vi "Phase Plots.vi"(4 "Impulse Positions":T3(array[cluster]) {"Amplitude offset" format="%.2f"}, 5 "Data Output":T4 {"Data Channels" format="%.2f"}, 7 "desacc":T1={"Threshold 1 [Acc]"=0.0, "Threshold 2 [% of TH1]"=0, "tolerance"=2, "Search WD "=0.05757575757575758, " always use TH2"=TRUE, "Range"=3.0303030303030303, "Max time"=50.0, "Min time"=1.0, "Velocity Threshold"=3.0303030303030303} {"Velocity Threshold" scale=0.0..5.0; "Range" scale=0.0..5.0; "Search WD" scale=0.0..0.3; "tolerance" scale=0.0..10.0; "Threshold 2 [% of TH1]" scale=0.0..100.0; "Threshold 1 [Acc]" scale=1.0..20000.0}) -> ()   [LabVIEW 2016]
uses:
  <vilib>/Analysis/baseanly.llb/Mean (DBL).vi
  comm/impulse/impulse functions.lvlib
  <vilib>/Analysis/NI_AALPro.lvlib
  <vilib>/Analysis/NI_AALBase.lvlib
panel:
  out "Angle Error":dbl format="%#_4g"
  out "Angle":dbl format="%#_4g"
  out "Slope":dbl
  out "Const":dbl
  out "Plane Equation":T2 {"Standard Deviation" format="%.6f"; "Z Slope" format="%.6f"; "Y Slope" format="%.6f"; "Offset" format="%.6f"}
  in  "Recalculate":bool
  in  "Horizontal Channel":u16(ring)=27
  in  "Vertical Channel":u16(ring)=27
  in  "Torsion Channel":u16(ring)=27
  in  "Fixed Absicca":bool
  in  "Fixed Ordinate":bool
  out "Phase Plot":cluster{dbl[], dbl[]}[](graph)
  in  "stop":bool
  in  "Off     Gain Inv         Absicca                         Off    Gain  Inv         Ordinate             Col  Sac    Plane          Data Range":T5(array[cluster])=[{"Color Box"=16777222, "Channel 1"=27, "inv 1"=FALSE, "Sac"=FALSE, "Offset 1"=0.0, "Gain 1"=1.0, "channel 2"=27, "Data From"=0, "Impulse Plane"=enum."Yaw", "inv 2"=FALSE, "Offset 2"=0.0, "Gain 2"=1.0}, {"Color Box"=3381759, "Channel 1"=5, "inv 1"=FALSE, "Sac"=FALSE, "Offset 1"=0.0, "Gain 1"=1.0, "channel 2"=27, "Data From"=0, "Impulse Plane"=enum."Yaw", "inv 2"=FALSE, "Offset 2"=0.0, "Gain 2"=1.0}] {"Gain 2" format="%.1f"; "Offset 2" format="%.1f"; "Data From" items=["All Data", "Impulse Data", "Peak Impulse Data"]; "Gain 1" format="%.1f"; "Offset 1" format="%.1f"}
  # "Vs."
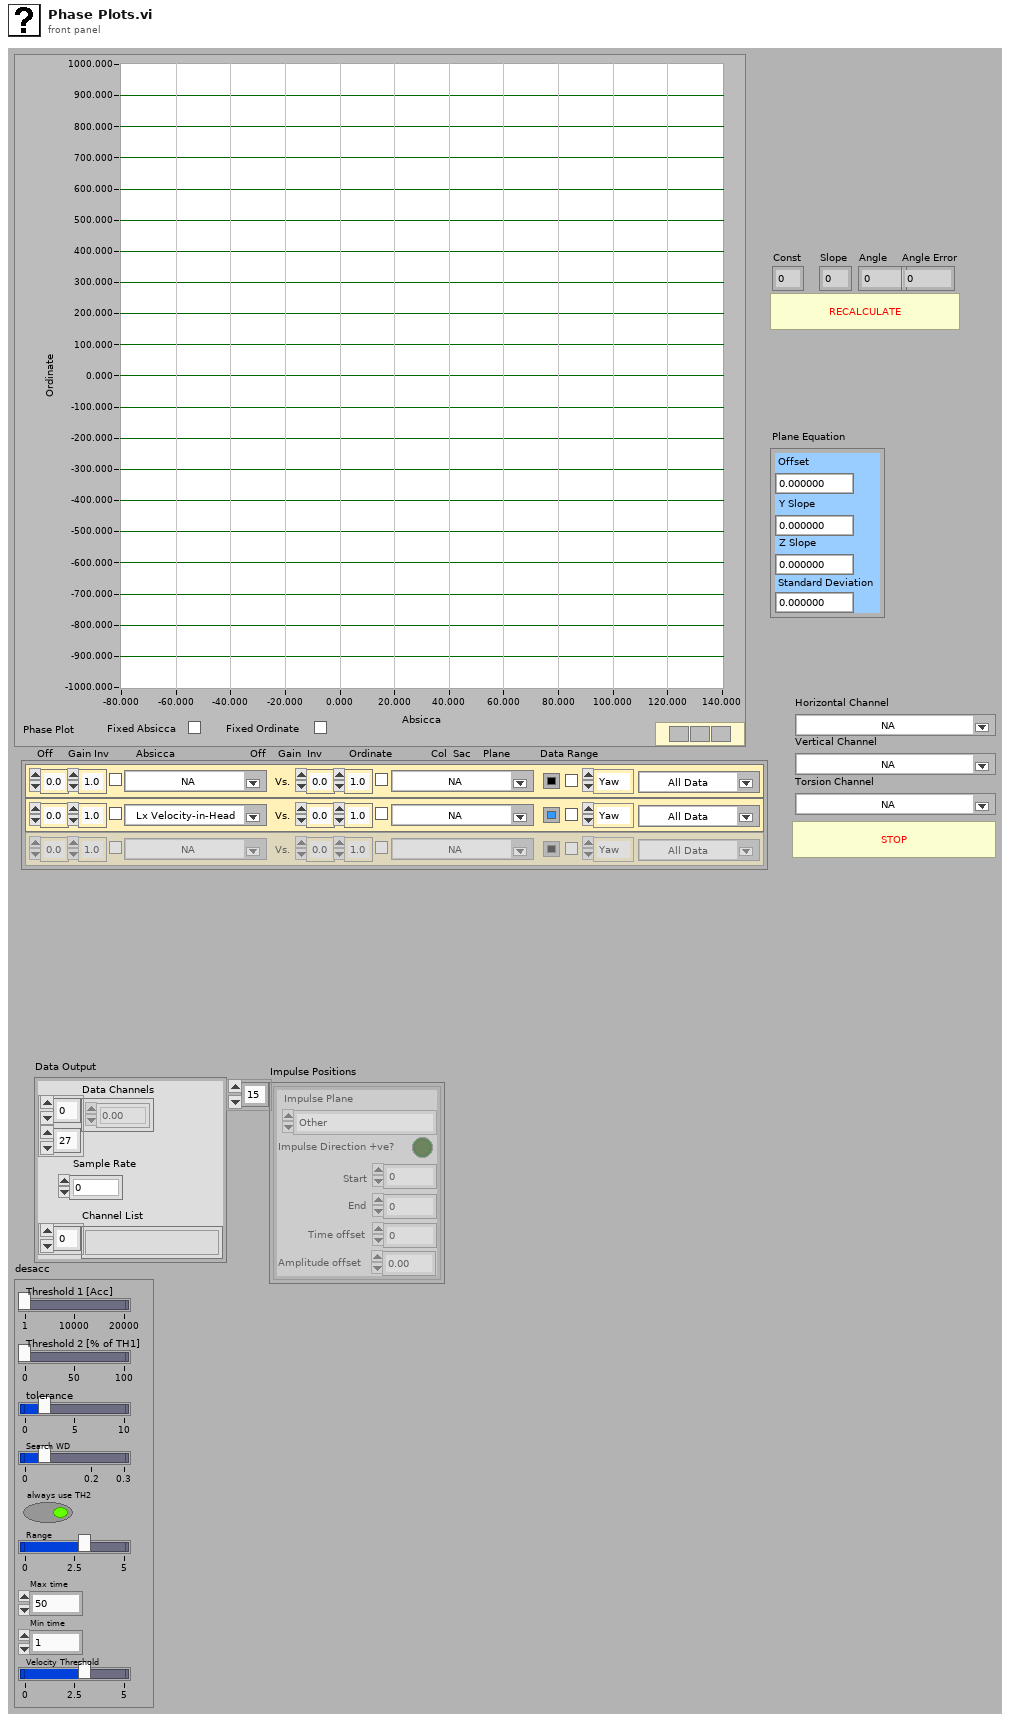
[diagram p1: front panel]
types:
  T1 = cluster{"Threshold 1 [Acc]":dbl, "Threshold 2 [% of TH1]":i32, "tolerance":i32, "Search WD ":dbl, " always use TH2":bool, "Range":dbl, "Max time":dbl, "Min time":dbl, "Velocity Threshold":dbl}
  T2 = cluster{"Offset":dbl, "Y Slope":dbl, "Z Slope":dbl, "Standard Deviation":dbl}
  T3 = cluster{"Start":i32, "End":i32, "Impulse Plane":enum16{"Other", "Yaw", "Pitch", "Roll", "LARP", "RALP"}, "Impulse Direction +ve?":bool, "Time offset":i32, "Amplitude offset":dbl}[]
  T4 = cluster{"Data Channels":dbl[][], "Sample Rate":i32, "Channel List":string[]}
  T5 = cluster{"Color Box":u32, "Channel 1":u16, "inv 1":bool, "Sac":bool, "Offset 1":dbl, "Gain 1":dbl, "channel 2":u16, "Data From":u16, "Impulse Plane":enum16{"Other", "Yaw", "Pitch", "Roll", "LARP", "RALP"}, "inv 2":bool, "Offset 2":dbl, "Gain 2":dbl}[]
  T6 = cluster{"Color Box":u32, "Boolean":bool, "List 1":u16, "Boolean 2":bool, "Boolean 3":bool, "Offset":dbl, "Gain":dbl}
  T7 = enum16{"Other", "Yaw", "Pitch", "Roll", "LARP", "RALP"}
  T8 = cluster{"Color Box":u32, "Boolean":bool, "List 1":u16, "Boolean 2":bool, "Boolean 3":bool, "Offset":dbl, "Gain":dbl}[]
  T9 = cluster{"Color Box":u32, "Channel 1":u16, "inv 1":bool, "Sac":bool, "Offset 1":dbl, "Gain 1":dbl, "channel 2":u16, "Data From":u16, "Impulse Plane":enum16{"Other", "Yaw", "Pitch", "Roll", "LARP", "RALP"}, "inv 2":bool, "Offset 2":dbl, "Gain 2":dbl}
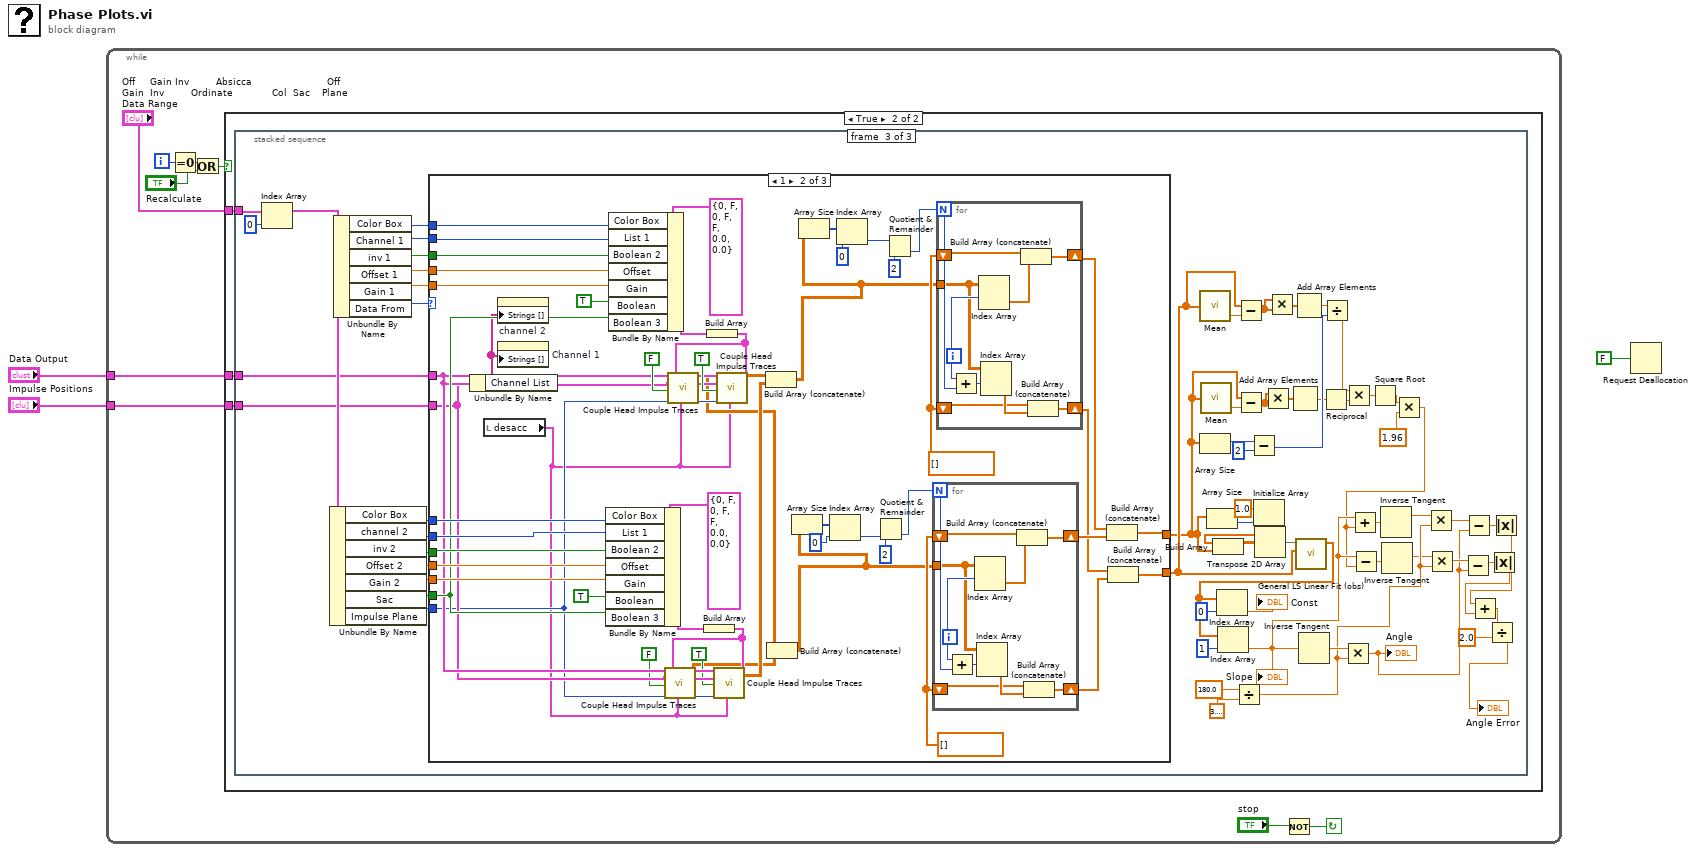
[diagram p0: block diagram]
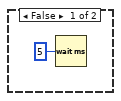
[diagram p2: hidden frame]
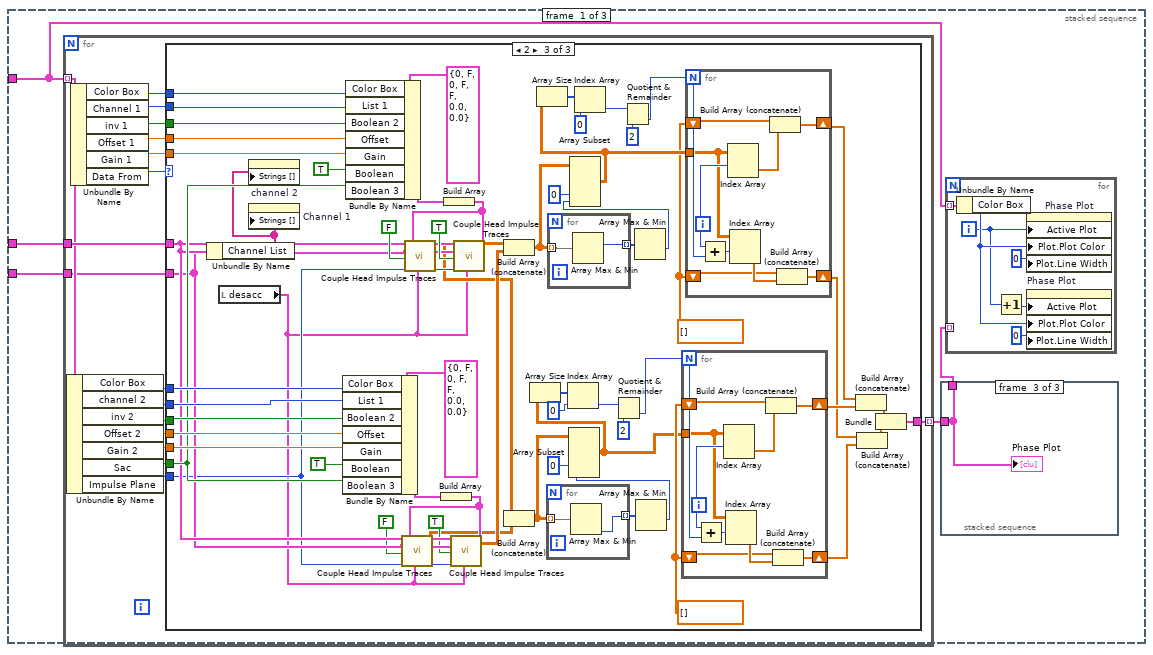
[diagram p3: hidden frame]
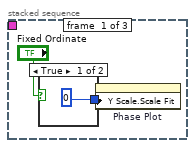
[diagram p4: hidden frame]
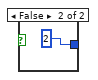
[diagram p5: hidden frame]
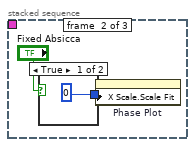
[diagram p6: hidden frame]
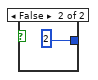
[diagram p7: hidden frame]
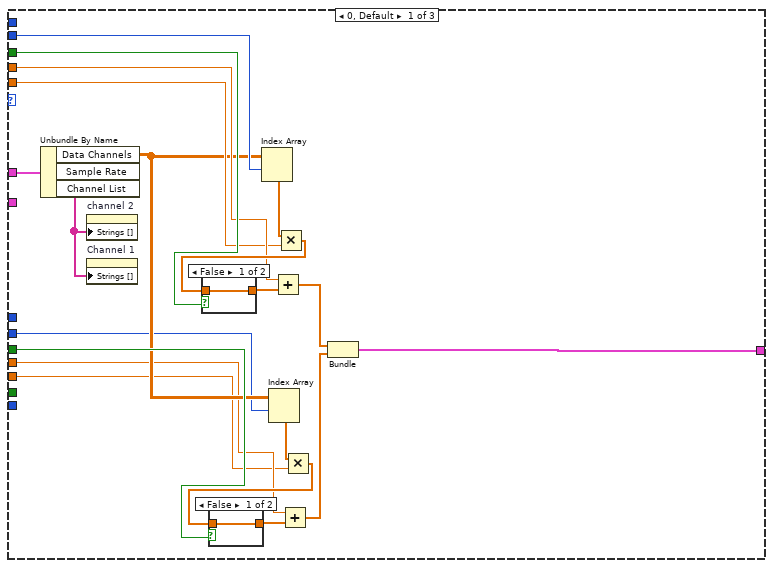
[diagram p8: hidden frame]
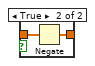
[diagram p9: hidden frame]
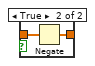
[diagram p10: hidden frame]
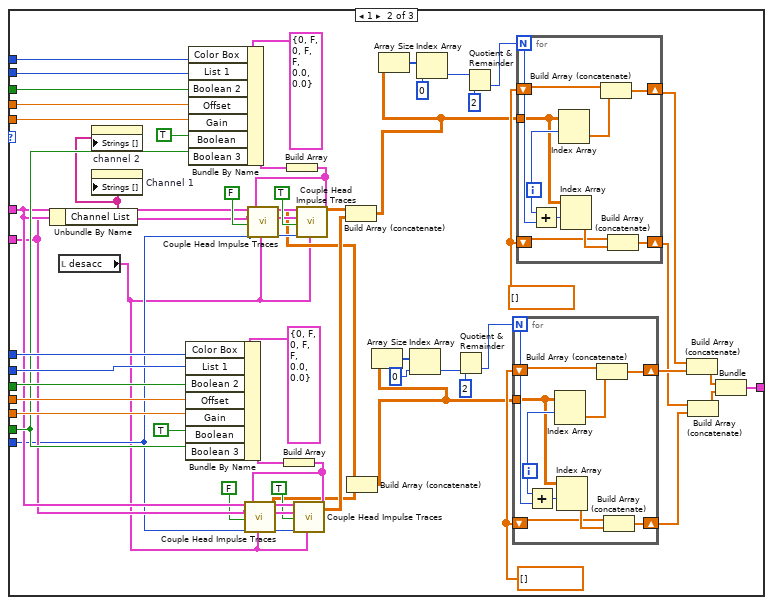
[diagram p11: hidden frame]
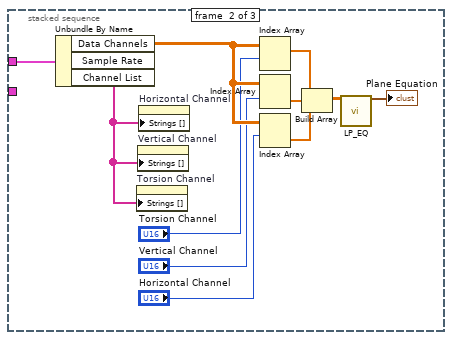
[diagram p12: hidden frame]
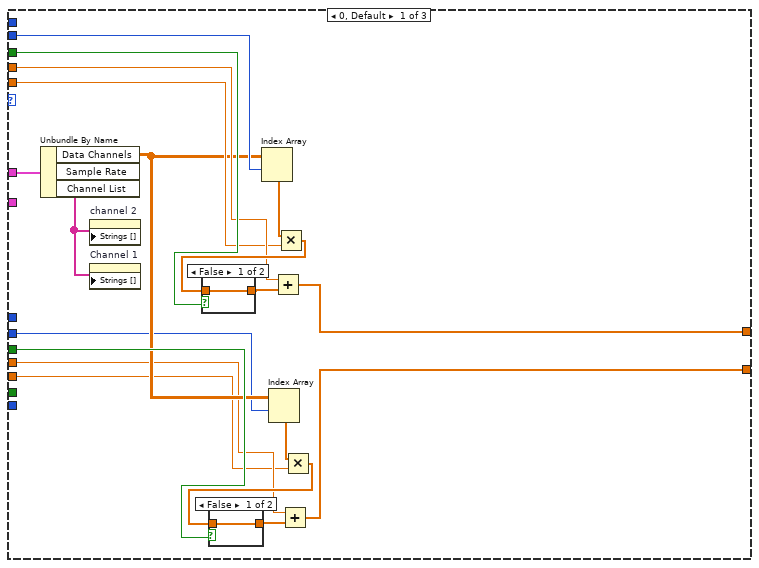
[diagram p13: hidden frame]
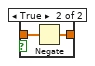
[diagram p14: hidden frame]
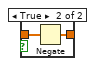
[diagram p15: hidden frame]
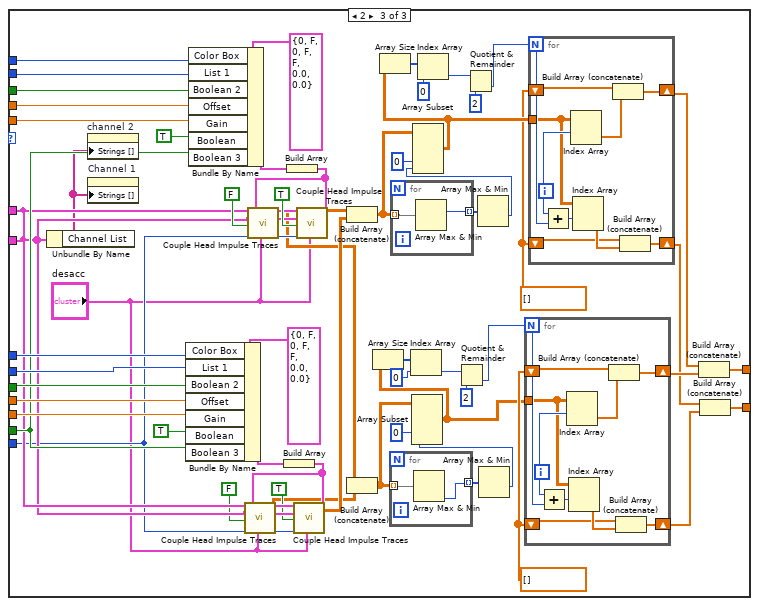
[diagram p16: hidden frame]
diagram:
  n1 = while {
    tunnel: "Data Output" -> [w10]
    tunnel: "Impulse Positions" -> [w9]
    i -> [w8]
    stop <- w11 continue-if-true
    n2 = Equal To 0?(x=w8) -> (x = 0?=w7:bool)
    n3 = Or(x=w7, y="Recalculate") -> (x .or. y?=w6:bool)
    n4 = case shown="True" w6 {
      tunnel: w10 -> [_ w16]
      tunnel: w9 -> [_ w15]
      tunnel: "Off     Gain Inv         Absicca                         Off    Gain  Inv         Ordinate             Col  Sac    Plane          Data Range" -> [_ w14]
      frame False {
        n5 = Wait (ms)(milliseconds to wait=u32 5) -> ()  [unwired: 1 out]
      }
      frame True {
        n6 = stacked-sequence {
          tunnel: w16 -> [w21 w239 w296]
          tunnel: w15 -> [w20 _ w297]
          tunnel: w14 -> [w19 _ w313]
          frame #0 {
            n7 = for {
              tunnel: w19 -> [w44] mode=indexing
              tunnel: w21 -> [w53]
              tunnel: w20 -> [w39]
              tunnel: [w37] -> w18 mode=indexing
              n8 = Unbundle By Name(w44) -> ("Color Box"=w38:u32, "channel 2"=w47:u16, "inv 2"=w48:bool, "Offset 2"=w46:dbl, "Gain 2"=w45:dbl, "Sac"=w41:bool, "Impulse Plane"=w40:T7)
              n9 = Unbundle By Name(w44) -> ("Color Box"=w43:u32, "Channel 1"=w52:u16, "inv 1"=w51:bool, "Offset 1"=w50:dbl, "Gain 1"=w49:dbl, "Data From"=w42:u16)
              n10 = case shown="2" w42 {
                tunnel: w53 -> [w73 w115 w196]
                tunnel: w52 -> [w69 w130 w211]
                tunnel: w51 -> [w68 w129 w210]
                tunnel: w50 -> [w67 w128 w209]
                tunnel: w49 -> [w66 w127 w208]
                tunnel: w48 -> [w63 w119 w200]
                tunnel: w47 -> [w61 w120 w201]
                tunnel: w46 -> [w60 w118 w199]
                tunnel: w45 -> [w59 w117 w198]
                tunnel: w43 -> [_ w87 w158]
                tunnel: w41 -> [_ w116 w197]
                tunnel: w40 -> [_ w111 w192]
                tunnel: w39 -> [_ w114 w195]
                tunnel: w38 -> [_ w121 w202]
                tunnel: [w54 w81 w154] -> w37
                frame 0, Default {
                  n11 = Unbundle By Name(w73) -> ("Data Channels"=w62:dbl[][], "Channel List"=w57:string[])  [unwired: 1 out]
                  n12 = property on="channel 2" class="Ring (strict)"("Strings []"=w57) -> ()  [unwired: 2 in, 2 out]
                  n13 = property on="Channel 1" class="Ring (strict)"("Strings []"=w57) -> ()  [unwired: 2 in, 2 out]
                  n14 = Index Array(array=w62, index (row)=w69) -> (element=w72:dbl[])  [unwired: 1 in]
                  n15 = Index Array(array=w62, index (row)=w61) -> (element=w58:dbl[])  [unwired: 1 in]
                  n16 = Multiply(x=w72, y=w66) -> (x*y=w71:dbl[])
                  n17 = case shown="False" w68 {
                    tunnel: w71 -> [w77 w79]
                    tunnel: [w77 w78] -> w70
                    frame False {
                    }
                    frame True {
                      n18 = Negate(x=w79) -> (-x=w78:dbl[])
                    }
                  }
                  n19 = Add(x=w67, y=w70) -> (x+y=w55:dbl[])
                  n20 = Multiply(x=w58, y=w59) -> (x*y=w64:dbl[])
                  n21 = case shown="False" w63 {
                    tunnel: w64 -> [w74 w76]
                    tunnel: [w74 w75] -> w65
                    frame False {
                    }
                    frame True {
                      n22 = Negate(x=w76) -> (-x=w75:dbl[])
                    }
                  }
                  n23 = Add(x=w60, y=w65) -> (x+y=w56:dbl[])
                  n24 = Bundle(w55, w56) -> (w54:cluster{dbl[], dbl[]})  [unwired: 1 in]
                }
                frame 1 {
                  w93 = dbl[] []
                  w96 = dbl[] []
                  n25 = Unbundle By Name(w115) -> ("Channel List"=w86:string[])
                  n26 = local read "desacc"() -> (w80:T1)
                  n27 = property on="channel 2" class="Ring (strict)"("Strings []"=w86) -> ()  [unwired: 2 in, 2 out]
                  n28 = property on="Channel 1" class="Ring (strict)"("Strings []"=w86) -> ()  [unwired: 2 in, 2 out]
                  n29 = Bundle By Name(cluster=T6 {"Color Box"=0, "Boolean"=FALSE, "List 1"=0, "Boolean 2"=FALSE, "Boolean 3"=FALSE, "Offset"=0.0, "Gain"=0.0} ("Cluster"), "Color Box"=w121, "List 1"=w120, "Boolean 2"=w119, "Offset"=w118, "Gain"=w117, "Boolean"=TRUE, "Boolean 3"=w116) -> (w123:T6)
                  n30 = Bundle By Name(cluster=T6 {"Color Box"=0, "Boolean"=FALSE, "List 1"=0, "Boolean 2"=FALSE, "Boolean 3"=FALSE, "Offset"=0.0, "Gain"=0.0} ("Cluster"), "Color Box"=w87, "List 1"=w130, "Boolean 2"=w129, "Offset"=w128, "Gain"=w127, "Boolean"=TRUE, "Boolean 3"=w116) -> (w125:T6)
                  n31 = Build Array(w123) -> (w113:T8)
                  n32 = call "Couple Head Impulse Traces.vi"("Data Input"=w115, "Impulse Positions"=w114, "Impulse Direction +ve?"=FALSE, "Impulse Plane"=w111, "Plot Selection 2"=w113, "desacc"=w80) -> ("Impulses"=w106:dbl[][])  [unwired: 10 in, 3 out]
                  n33 = Build Array(w125) -> (w124:T8)
                  n34 = call "Couple Head Impulse Traces.vi"("Data Input"=w115, "Impulse Positions"=w114, "Impulse Direction +ve?"=FALSE, "Impulse Plane"=w111, "Plot Selection 2"=w124, "desacc"=w80) -> ("Impulses"=w105:dbl[][])  [unwired: 10 in, 3 out]
                  n35 = call "Couple Head Impulse Traces.vi"("Data Input"=w115, "Impulse Positions"=w114, "Impulse Direction +ve?"=TRUE, "Impulse Plane"=w111, "Plot Selection 2"=w113, "desacc"=w80) -> ("Impulses"=w107:dbl[][])  [unwired: 10 in, 3 out]
                  n36 = call "Couple Head Impulse Traces.vi"("Data Input"=w115, "Impulse Positions"=w114, "Impulse Direction +ve?"=TRUE, "Impulse Plane"=w111, "Plot Selection 2"=w124, "desacc"=w80) -> ("Impulses"=w108:dbl[][])  [unwired: 10 in, 3 out]
                  n37 = Build Array (concatenate)(w108, w107) -> (w84:dbl[][])
                  n38 = Build Array (concatenate)(w105, w106) -> (w85:dbl[][])
                  n39 = Array Size(array=w85) -> (size(s)=w100:i32[])
                  n40 = Array Size(array=w84) -> (size(s)=w103:i32[])
                  n41 = Index Array(array=w100, index=0) -> (element=w94:i32)
                  n42 = Index Array(array=w103, index=0) -> (element=w99:i32)
                  n43 = Quotient & Remainder(x=w94, y=2) -> (floor(x/y)=w92:i32)  [unwired: 1 out]
                  n44 = Quotient & Remainder(x=w99, y=2) -> (floor(x/y)=w97:i32)  [unwired: 1 out]
                  n45 = for {
                    N: w92 -> [w140]
                    tunnel: w85 -> [w133]
                    shift-right: [w138] -> w90
                    shift-left: w93 -> [w137]
                    shift-right: [w136] -> w89
                    shift-left: w93 -> [w134]
                    i -> [w142]
                    n46 = Add(x=w142, y=w140) -> (x+y=w141:i32)
                    n47 = Index Array(array=w133, index (row)=w142) -> (element=w139:dbl[])  [unwired: 1 in]
                    n48 = Index Array(array=w133, index (row)=w141) -> (element=w135:dbl[])  [unwired: 1 in]
                    n49 = Build Array (concatenate)(w137, w139) -> (w138:dbl[])
                    n50 = Build Array (concatenate)(w134, w135) -> (w136:dbl[])
                  }
                  n51 = for {
                    N: w97 -> [w150]
                    tunnel: w84 -> [w143]
                    shift-right: [w148] -> w91
                    shift-left: w96 -> [w147]
                    shift-right: [w146] -> w88
                    shift-left: w96 -> [w144]
                    i -> [w152]
                    n52 = Add(x=w152, y=w150) -> (x+y=w151:i32)
                    n53 = Index Array(array=w143, index (row)=w152) -> (element=w149:dbl[])  [unwired: 1 in]
                    n54 = Index Array(array=w143, index (row)=w151) -> (element=w145:dbl[])  [unwired: 1 in]
                    n55 = Build Array (concatenate)(w147, w149) -> (w148:dbl[])
                    n56 = Build Array (concatenate)(w144, w145) -> (w146:dbl[])
                  }
                  n57 = Build Array (concatenate)(w91, w90) -> (w83:dbl[])
                  n58 = Build Array (concatenate)(w88, w89) -> (w82:dbl[])
                  n59 = Bundle(w83, w82) -> (w81:cluster{dbl[], dbl[]})  [unwired: 1 in]
                }
                frame 2 {
                  w165 = dbl[] []
                  w168 = dbl[] []
                  n60 = Unbundle By Name(w196) -> ("Channel List"=w157:string[])
                  n61 = local read "desacc"() -> (w153:T1)
                  n62 = property on="channel 2" class="Ring (strict)"("Strings []"=w157) -> ()  [unwired: 2 in, 2 out]
                  n63 = property on="Channel 1" class="Ring (strict)"("Strings []"=w157) -> ()  [unwired: 2 in, 2 out]
                  n64 = Bundle By Name(cluster=T6 {"Color Box"=0, "Boolean"=FALSE, "List 1"=0, "Boolean 2"=FALSE, "Boolean 3"=FALSE, "Offset"=0.0, "Gain"=0.0} ("Cluster"), "Color Box"=w202, "List 1"=w201, "Boolean 2"=w200, "Offset"=w199, "Gain"=w198, "Boolean"=TRUE, "Boolean 3"=w197) -> (w204:T6)
                  n65 = Bundle By Name(cluster=T6 {"Color Box"=0, "Boolean"=FALSE, "List 1"=0, "Boolean 2"=FALSE, "Boolean 3"=FALSE, "Offset"=0.0, "Gain"=0.0} ("Cluster"), "Color Box"=w158, "List 1"=w211, "Boolean 2"=w210, "Offset"=w209, "Gain"=w208, "Boolean"=TRUE, "Boolean 3"=w197) -> (w206:T6)
                  n66 = Build Array(w204) -> (w194:T8)
                  n67 = call "Couple Head Impulse Traces.vi"("Data Input"=w196, "Impulse Positions"=w195, "Impulse Direction +ve?"=FALSE, "Impulse Plane"=w192, "Plot Selection 2"=w194, "desacc"=w153) -> ("Impulses"=w183:dbl[][])  [unwired: 10 in, 3 out]
                  n68 = Build Array(w206) -> (w205:T8)
                  n69 = call "Couple Head Impulse Traces.vi"("Data Input"=w196, "Impulse Positions"=w195, "Impulse Direction +ve?"=FALSE, "Impulse Plane"=w192, "Plot Selection 2"=w205, "desacc"=w153) -> ("Impulses"=w182:dbl[][])  [unwired: 10 in, 3 out]
                  n70 = call "Couple Head Impulse Traces.vi"("Data Input"=w196, "Impulse Positions"=w195, "Impulse Direction +ve?"=TRUE, "Impulse Plane"=w192, "Plot Selection 2"=w194, "desacc"=w153) -> ("Impulses"=w187:dbl[][])  [unwired: 10 in, 3 out]
                  n71 = call "Couple Head Impulse Traces.vi"("Data Input"=w196, "Impulse Positions"=w195, "Impulse Direction +ve?"=TRUE, "Impulse Plane"=w192, "Plot Selection 2"=w205, "desacc"=w153) -> ("Impulses"=w188:dbl[][])  [unwired: 10 in, 3 out]
                  n72 = Build Array (concatenate)(w188, w187) -> (w186:dbl[][])
                  n73 = Build Array (concatenate)(w182, w183) -> (w185:dbl[][])
                  n74 = for {
                    tunnel: w185 -> [w235] mode=indexing
                    tunnel: [w234] -> w184 mode=indexing
                    n75 = Array Max & Min(array=w235) -> (min index (indices)=w234:i32)  [unwired: 3 out]
                  }
                  n76 = for {
                    tunnel: w186 -> [w237] mode=indexing
                    tunnel: [w236] -> w189 mode=indexing
                    n77 = Array Max & Min(array=w237) -> (max index (indices)=w236:i32)  [unwired: 3 out]
                  }
                  n78 = Array Max & Min(array=w189) -> (min value=w179:i32)  [unwired: 3 out]
                  n79 = Array Subset(array=w186, index (col)=0 ("index"), length (col)=w179) -> (w169:dbl[][])  [unwired: 2 in]
                  n80 = Array Size(array=w169) -> (size(s)=w176:i32[])
                  n81 = Index Array(array=w176, index=0) -> (element=w172:i32)
                  n82 = Quotient & Remainder(x=w172, y=2) -> (floor(x/y)=w170:i32)  [unwired: 1 out]
                  n83 = Array Max & Min(array=w184) -> (min value=w177:i32)  [unwired: 3 out]
                  n84 = Array Subset(array=w185, index (col)=0 ("index"), length (col)=w177) -> (w163:dbl[][])  [unwired: 2 in]
                  n85 = Array Size(array=w163) -> (size(s)=w173:i32[])
                  n86 = Index Array(array=w173, index=0) -> (element=w166:i32)
                  n87 = Quotient & Remainder(x=w166, y=2) -> (floor(x/y)=w164:i32)  [unwired: 1 out]
                  n88 = for {
                    N: w164 -> [w221]
                    tunnel: w163 -> [w214]
                    shift-right: [w219] -> w161
                    shift-left: w165 -> [w218]
                    shift-right: [w217] -> w160
                    shift-left: w165 -> [w215]
                    i -> [w223]
                    n89 = Add(x=w223, y=w221) -> (x+y=w222:i32)
                    n90 = Index Array(array=w214, index (row)=w223) -> (element=w220:dbl[])  [unwired: 1 in]
                    n91 = Index Array(array=w214, index (row)=w222) -> (element=w216:dbl[])  [unwired: 1 in]
                    n92 = Build Array (concatenate)(w218, w220) -> (w219:dbl[])
                    n93 = Build Array (concatenate)(w215, w216) -> (w217:dbl[])
                  }
                  n94 = for {
                    N: w170 -> [w231]
                    tunnel: w169 -> [w224]
                    shift-right: [w229] -> w162
                    shift-left: w168 -> [w228]
                    shift-right: [w227] -> w159
                    shift-left: w168 -> [w225]
                    i -> [w233]
                    n95 = Add(x=w233, y=w231) -> (x+y=w232:i32)
                    n96 = Index Array(array=w224, index (row)=w233) -> (element=w230:dbl[])  [unwired: 1 in]
                    n97 = Index Array(array=w224, index (row)=w232) -> (element=w226:dbl[])  [unwired: 1 in]
                    n98 = Build Array (concatenate)(w228, w230) -> (w229:dbl[])
                    n99 = Build Array (concatenate)(w225, w226) -> (w227:dbl[])
                  }
                  n100 = Build Array (concatenate)(w162, w161) -> (w155:dbl[])
                  n101 = Build Array (concatenate)(w159, w160) -> (w156:dbl[])
                  n102 = Bundle(w155, w156) -> (w154:cluster{dbl[], dbl[]})  [unwired: 1 in]
                }
              }
            }
            n103 = stacked-sequence {
              tunnel: w18 -> [_ _ w30]
              tunnel: [_ _ w30] -> w17
              frame #0 {
                n104 = case shown="True" "Fixed Ordinate" {
                  tunnel: [u8 0 ("Y Scale.Scale Fit") u8 2 ("Y Scale.Scale Fit")] -> w23
                  frame True {
                  }
                  frame False {
                  }
                }
                n105 = property on="Phase Plot" class="XYGraph (strict)"("Y Scale.Scale Fit"=w23) -> ()  [unwired: 2 in, 2 out]
              }
              frame #1 {
                n106 = case shown="True" "Fixed Absicca" {
                  tunnel: [u8 0 ("Y Scale.Scale Fit") u8 2 ("Y Scale.Scale Fit")] -> w27
                  frame True {
                  }
                  frame False {
                  }
                }
                n107 = property on="Phase Plot" class="XYGraph (strict)"("X Scale.Scale Fit"=w27) -> ()  [unwired: 2 in, 2 out]
              }
              frame #2 {
                "Phase Plot" <- w30
              }
            }
            n108 = for {
              tunnel: w19 -> [w36] mode=indexing
              tunnel: w17 -> [_] mode=indexing
              i -> [w31]
              n109 = Unbundle By Name(w36) -> ("Color Box"=w32:u32)
              n110 = Increment(x=w31) -> (x+1=w34:i32)
              n111 = property on="Phase Plot" class="XYGraph (strict)"("Active Plot"=w31, "Plot.Plot Color"=w32, "Plot.Line Width"=u8 0) -> ()  [unwired: 2 in, 2 out]
              n112 = property on="Phase Plot" class="XYGraph (strict)"("Active Plot"=w34, "Plot.Plot Color"=w32, "Plot.Line Width"=u8 0) -> ()  [unwired: 2 in, 2 out]
            }
          }
          frame #1 {
            n113 = Unbundle By Name(w239) -> ("Data Channels"=w247:dbl[][], "Channel List"=w248:string[])  [unwired: 1 out]
            n114 = property on="Torsion Channel" class="Ring (strict)"("Strings []"=w248) -> ()  [unwired: 2 in, 2 out]
            n115 = property on="Vertical Channel" class="Ring (strict)"("Strings []"=w248) -> ()  [unwired: 2 in, 2 out]
            n116 = property on="Horizontal Channel" class="Ring (strict)"("Strings []"=w248) -> ()  [unwired: 2 in, 2 out]
            n117 = Index Array(array=w247, index (row)="Torsion Channel") -> (element=w245:dbl[])  [unwired: 1 in]
            n118 = Index Array(array=w247, index (row)="Vertical Channel") -> (element=w244:dbl[])  [unwired: 1 in]
            n119 = Index Array(array=w247, index (row)="Horizontal Channel") -> (element=w243:dbl[])  [unwired: 1 in]
            n120 = Build Array(w245, w244, w243) -> (w242:dbl[][])
            n121 = call "LP_EQ.VI"("Rotation Vectors"=w242) -> ("Plane Equation"=→"Plane Equation":T2)  [unwired: 17 in, 1 out]
          }
          frame #2 {
            n122 = Index Array(array=w313, index=0) -> (element=w298:T9)
            n123 = Unbundle By Name(w298) -> ("Color Box"=w299:u32, "channel 2"=w306:u16, "inv 2"=w307:bool, "Offset 2"=w305:dbl, "Gain 2"=w304:dbl, "Sac"=w301:bool, "Impulse Plane"=w300:T7)
            n124 = Unbundle By Name(w298) -> ("Color Box"=w303:u32, "Channel 1"=w311:u16, "inv 1"=w310:bool, "Offset 1"=w309:dbl, "Gain 1"=w308:dbl, "Data From"=w302:u16)
            n125 = case shown="1" w302 {
              tunnel: w296 -> [w332 w373 w453]
              tunnel: w311 -> [w328 w388 w468]
              tunnel: w310 -> [w327 w387 w467]
              tunnel: w309 -> [w326 w386 w466]
              tunnel: w308 -> [w325 w385 w465]
              tunnel: w307 -> [w322 w377 w457]
              tunnel: w306 -> [w320 w378 w458]
              tunnel: w305 -> [w319 w376 w456]
              tunnel: w304 -> [w318 w375 w455]
              tunnel: w303 -> [_ w345 w415]
              tunnel: w301 -> [_ w374 w454]
              tunnel: w300 -> [_ w369 w449]
              tunnel: w297 -> [_ w372 w452]
              tunnel: w299 -> [_ w379 w459]
              tunnel: [w315 w341 w413] -> w269
              tunnel: [w314 w340 w412] -> w270
              frame 0, Default {
                n126 = Unbundle By Name(w332) -> ("Data Channels"=w321:dbl[][], "Channel List"=w316:string[])  [unwired: 1 out]
                n127 = property on="channel 2" class="Ring (strict)"("Strings []"=w316) -> ()  [unwired: 2 in, 2 out]
                n128 = property on="Channel 1" class="Ring (strict)"("Strings []"=w316) -> ()  [unwired: 2 in, 2 out]
                n129 = Index Array(array=w321, index (row)=w328) -> (element=w331:dbl[])  [unwired: 1 in]
                n130 = Index Array(array=w321, index (row)=w320) -> (element=w317:dbl[])  [unwired: 1 in]
                n131 = Multiply(x=w331, y=w325) -> (x*y=w330:dbl[])
                n132 = case shown="False" w327 {
                  tunnel: w330 -> [w336 w338]
                  tunnel: [w336 w337] -> w329
                  frame False {
                  }
                  frame True {
                    n133 = Negate(x=w338) -> (-x=w337:dbl[])
                  }
                }
                n134 = Add(x=w326, y=w329) -> (x+y=w315:dbl[])
                n135 = Multiply(x=w317, y=w318) -> (x*y=w323:dbl[])
                n136 = case shown="False" w322 {
                  tunnel: w323 -> [w333 w335]
                  tunnel: [w333 w334] -> w324
                  frame False {
                  }
                  frame True {
                    n137 = Negate(x=w335) -> (-x=w334:dbl[])
                  }
                }
                n138 = Add(x=w319, y=w324) -> (x+y=w314:dbl[])
              }
              frame 1 {
                w351 = dbl[] []
                w354 = dbl[] []
                n139 = Unbundle By Name(w373) -> ("Channel List"=w342:string[])
                n140 = local read "desacc"() -> (w339:T1)
                n141 = property on="channel 2" class="Ring (strict)"("Strings []"=w342) -> ()  [unwired: 2 in, 2 out]
                n142 = property on="Channel 1" class="Ring (strict)"("Strings []"=w342) -> ()  [unwired: 2 in, 2 out]
                n143 = Bundle By Name(cluster=T6 {"Color Box"=0, "Boolean"=FALSE, "List 1"=0, "Boolean 2"=FALSE, "Boolean 3"=FALSE, "Offset"=0.0, "Gain"=0.0} ("Cluster"), "Color Box"=w379, "List 1"=w378, "Boolean 2"=w377, "Offset"=w376, "Gain"=w375, "Boolean"=TRUE, "Boolean 3"=w374) -> (w381:T6)
                n144 = Bundle By Name(cluster=T6 {"Color Box"=0, "Boolean"=FALSE, "List 1"=0, "Boolean 2"=FALSE, "Boolean 3"=FALSE, "Offset"=0.0, "Gain"=0.0} ("Cluster"), "Color Box"=w345, "List 1"=w388, "Boolean 2"=w387, "Offset"=w386, "Gain"=w385, "Boolean"=TRUE, "Boolean 3"=w374) -> (w383:T6)
                n145 = Build Array(w381) -> (w371:T8)
                n146 = call "Couple Head Impulse Traces.vi"("Data Input"=w373, "Impulse Positions"=w372, "Impulse Direction +ve?"=FALSE, "Impulse Plane"=w369, "Plot Selection 2"=w371, "desacc"=w339) -> ("Impulses"=w364:dbl[][])  [unwired: 10 in, 3 out]
                n147 = Build Array(w383) -> (w382:T8)
                n148 = call "Couple Head Impulse Traces.vi"("Data Input"=w373, "Impulse Positions"=w372, "Impulse Direction +ve?"=FALSE, "Impulse Plane"=w369, "Plot Selection 2"=w382, "desacc"=w339) -> ("Impulses"=w363:dbl[][])  [unwired: 10 in, 3 out]
                n149 = call "Couple Head Impulse Traces.vi"("Data Input"=w373, "Impulse Positions"=w372, "Impulse Direction +ve?"=TRUE, "Impulse Plane"=w369, "Plot Selection 2"=w371, "desacc"=w339) -> ("Impulses"=w365:dbl[][])  [unwired: 10 in, 3 out]
                n150 = call "Couple Head Impulse Traces.vi"("Data Input"=w373, "Impulse Positions"=w372, "Impulse Direction +ve?"=TRUE, "Impulse Plane"=w369, "Plot Selection 2"=w382, "desacc"=w339) -> ("Impulses"=w366:dbl[][])  [unwired: 10 in, 3 out]
                n151 = Build Array (concatenate)(w366, w365) -> (w343:dbl[][])
                n152 = Build Array (concatenate)(w363, w364) -> (w344:dbl[][])
                n153 = Array Size(array=w344) -> (size(s)=w358:i32[])
                n154 = Array Size(array=w343) -> (size(s)=w361:i32[])
                n155 = Index Array(array=w358, index=0) -> (element=w352:i32)
                n156 = Index Array(array=w361, index=0) -> (element=w357:i32)
                n157 = Quotient & Remainder(x=w352, y=2) -> (floor(x/y)=w350:i32)  [unwired: 1 out]
                n158 = Quotient & Remainder(x=w357, y=2) -> (floor(x/y)=w355:i32)  [unwired: 1 out]
                n159 = for {
                  N: w350 -> [w398]
                  tunnel: w344 -> [w391]
                  shift-right: [w396] -> w348
                  shift-left: w351 -> [w395]
                  shift-right: [w394] -> w347
                  shift-left: w351 -> [w392]
                  i -> [w400]
                  n160 = Add(x=w400, y=w398) -> (x+y=w399:i32)
                  n161 = Index Array(array=w391, index (row)=w400) -> (element=w397:dbl[])  [unwired: 1 in]
                  n162 = Index Array(array=w391, index (row)=w399) -> (element=w393:dbl[])  [unwired: 1 in]
                  n163 = Build Array (concatenate)(w395, w397) -> (w396:dbl[])
                  n164 = Build Array (concatenate)(w392, w393) -> (w394:dbl[])
                }
                n165 = for {
                  N: w355 -> [w408]
                  tunnel: w343 -> [w401]
                  shift-right: [w406] -> w349
                  shift-left: w354 -> [w405]
                  shift-right: [w404] -> w346
                  shift-left: w354 -> [w402]
                  i -> [w410]
                  n166 = Add(x=w410, y=w408) -> (x+y=w409:i32)
                  n167 = Index Array(array=w401, index (row)=w410) -> (element=w407:dbl[])  [unwired: 1 in]
                  n168 = Index Array(array=w401, index (row)=w409) -> (element=w403:dbl[])  [unwired: 1 in]
                  n169 = Build Array (concatenate)(w405, w407) -> (w406:dbl[])
                  n170 = Build Array (concatenate)(w402, w403) -> (w404:dbl[])
                }
                n171 = Build Array (concatenate)(w349, w348) -> (w341:dbl[])
                n172 = Build Array (concatenate)(w346, w347) -> (w340:dbl[])
              }
              frame 2 {
                w422 = dbl[] []
                w425 = dbl[] []
                n173 = Unbundle By Name(w453) -> ("Channel List"=w414:string[])
                n174 = property on="channel 2" class="Ring (strict)"("Strings []"=w414) -> ()  [unwired: 2 in, 2 out]
                n175 = property on="Channel 1" class="Ring (strict)"("Strings []"=w414) -> ()  [unwired: 2 in, 2 out]
                n176 = Bundle By Name(cluster=T6 {"Color Box"=0, "Boolean"=FALSE, "List 1"=0, "Boolean 2"=FALSE, "Boolean 3"=FALSE, "Offset"=0.0, "Gain"=0.0} ("Cluster"), "Color Box"=w459, "List 1"=w458, "Boolean 2"=w457, "Offset"=w456, "Gain"=w455, "Boolean"=TRUE, "Boolean 3"=w454) -> (w461:T6)
                n177 = Bundle By Name(cluster=T6 {"Color Box"=0, "Boolean"=FALSE, "List 1"=0, "Boolean 2"=FALSE, "Boolean 3"=FALSE, "Offset"=0.0, "Gain"=0.0} ("Cluster"), "Color Box"=w415, "List 1"=w468, "Boolean 2"=w467, "Offset"=w466, "Gain"=w465, "Boolean"=TRUE, "Boolean 3"=w454) -> (w463:T6)
                n178 = Build Array(w461) -> (w451:T8)
                n179 = call "Couple Head Impulse Traces.vi"("Data Input"=w453, "Impulse Positions"=w452, "Impulse Direction +ve?"=FALSE, "Impulse Plane"=w449, "Plot Selection 2"=w451, "desacc"="desacc") -> ("Impulses"=w440:dbl[][])  [unwired: 10 in, 3 out]
                n180 = Build Array(w463) -> (w462:T8)
                n181 = call "Couple Head Impulse Traces.vi"("Data Input"=w453, "Impulse Positions"=w452, "Impulse Direction +ve?"=FALSE, "Impulse Plane"=w449, "Plot Selection 2"=w462, "desacc"="desacc") -> ("Impulses"=w439:dbl[][])  [unwired: 10 in, 3 out]
                n182 = call "Couple Head Impulse Traces.vi"("Data Input"=w453, "Impulse Positions"=w452, "Impulse Direction +ve?"=TRUE, "Impulse Plane"=w449, "Plot Selection 2"=w451, "desacc"="desacc") -> ("Impulses"=w444:dbl[][])  [unwired: 10 in, 3 out]
                n183 = call "Couple Head Impulse Traces.vi"("Data Input"=w453, "Impulse Positions"=w452, "Impulse Direction +ve?"=TRUE, "Impulse Plane"=w449, "Plot Selection 2"=w462, "desacc"="desacc") -> ("Impulses"=w445:dbl[][])  [unwired: 10 in, 3 out]
                n184 = Build Array (concatenate)(w445, w444) -> (w443:dbl[][])
                n185 = Build Array (concatenate)(w439, w440) -> (w442:dbl[][])
                n186 = for {
                  tunnel: w442 -> [w492] mode=indexing
                  tunnel: [w491] -> w441 mode=indexing
                  n187 = Array Max & Min(array=w492) -> (min index (indices)=w491:i32)  [unwired: 3 out]
                }
                n188 = for {
                  tunnel: w443 -> [w494] mode=indexing
                  tunnel: [w493] -> w446 mode=indexing
                  n189 = Array Max & Min(array=w494) -> (max index (indices)=w493:i32)  [unwired: 3 out]
                }
                n190 = Array Max & Min(array=w446) -> (min value=w436:i32)  [unwired: 3 out]
                n191 = Array Subset(array=w443, index (col)=0 ("index"), length (col)=w436) -> (w426:dbl[][])  [unwired: 2 in]
                n192 = Array Size(array=w426) -> (size(s)=w433:i32[])
                n193 = Index Array(array=w433, index=0) -> (element=w429:i32)
                n194 = Quotient & Remainder(x=w429, y=2) -> (floor(x/y)=w427:i32)  [unwired: 1 out]
                n195 = Array Max & Min(array=w441) -> (min value=w434:i32)  [unwired: 3 out]
                n196 = Array Subset(array=w442, index (col)=0 ("index"), length (col)=w434) -> (w420:dbl[][])  [unwired: 2 in]
                n197 = Array Size(array=w420) -> (size(s)=w430:i32[])
                n198 = Index Array(array=w430, index=0) -> (element=w423:i32)
                n199 = Quotient & Remainder(x=w423, y=2) -> (floor(x/y)=w421:i32)  [unwired: 1 out]
                n200 = for {
                  N: w421 -> [w478]
                  tunnel: w420 -> [w471]
                  shift-right: [w476] -> w418
                  shift-left: w422 -> [w475]
                  shift-right: [w474] -> w417
                  shift-left: w422 -> [w472]
                  i -> [w480]
                  n201 = Add(x=w480, y=w478) -> (x+y=w479:i32)
                  n202 = Index Array(array=w471, index (row)=w480) -> (element=w477:dbl[])  [unwired: 1 in]
                  n203 = Index Array(array=w471, index (row)=w479) -> (element=w473:dbl[])  [unwired: 1 in]
                  n204 = Build Array (concatenate)(w475, w477) -> (w476:dbl[])
                  n205 = Build Array (concatenate)(w472, w473) -> (w474:dbl[])
                }
                n206 = for {
                  N: w427 -> [w488]
                  tunnel: w426 -> [w481]
                  shift-right: [w486] -> w419
                  shift-left: w425 -> [w485]
                  shift-right: [w484] -> w416
                  shift-left: w425 -> [w482]
                  i -> [w490]
                  n207 = Add(x=w490, y=w488) -> (x+y=w489:i32)
                  n208 = Index Array(array=w481, index (row)=w490) -> (element=w487:dbl[])  [unwired: 1 in]
                  n209 = Index Array(array=w481, index (row)=w489) -> (element=w483:dbl[])  [unwired: 1 in]
                  n210 = Build Array (concatenate)(w485, w487) -> (w486:dbl[])
                  n211 = Build Array (concatenate)(w482, w483) -> (w484:dbl[])
                }
                n212 = Build Array (concatenate)(w419, w418) -> (w413:dbl[])
                n213 = Build Array (concatenate)(w416, w417) -> (w412:dbl[])
              }
            }
            n214 = call-poly <vilib>:"Mean.vi"("X"=w270) -> ("mean"=w286:dbl)  [unwired: 1 out]
            n215 = Array Size(array=w269) -> (size(s)=w284:i32)
            n216 = call-poly <vilib>:"Mean.vi"("X"=w269) -> ("mean"=w285:dbl)  [unwired: 1 out]
            n217 = Array Size(array=w269) -> (size(s)=w295:i32)
            n218 = Divide(x=180.0, y=3.141592653589793) -> (x/y=w261:dbl)
            n219 = Subtract(x=w270, y=w286) -> (x-y=w282:dbl[])
            n220 = Subtract(x=w269, y=w285) -> (x-y=w281:dbl[])
            n221 = Subtract(x=w284, y=2) -> (x-y=w279:i32)
            n222 = Initialize Array(1.0 ("element"), w295) -> (w293:dbl[])
            n223 = Build Array(w293, w269) -> (w292:dbl[][])
            n224 = Transpose 2D Array(2D array=w292) -> (transposed array=w287:dbl[][])
            n225 = Multiply(x=w281, y=w281) -> (x*y=w277:dbl[])
            n226 = Multiply(x=w282, y=w282) -> (x*y=w280:dbl[])
            n227 = Add Array Elements(numeric array=w277) -> (sum=w276:dbl)
            n228 = Add Array Elements(numeric array=w280) -> (sum=w278:dbl)
            n229 = call <vilib>:"General LS Linear Fit (obs).vi"("H"=w287, "Y"=w270) -> ("Coefficients"=w291:dbl[])  [unwired: 3 in, 4 out]
            n230 = Index Array(array=w291, index=0) -> (element=→"Const":dbl)
            n231 = Index Array(array=w291, index=1) -> (element=w265:dbl)
            "Slope" <- w265
            n232 = Inverse Tangent(1:w265) -> (0:w268:dbl)
            n233 = Reciprocal(x=w276) -> (1/x=w275:dbl)
            n234 = Divide(x=w278, y=w279) -> (x/y=w274:dbl)
            n235 = Multiply(x=w268, y=w261) -> (x*y=w256:dbl)
            "Angle" <- w256
            n236 = Multiply(x=w274, y=w275) -> (x*y=w273:dbl)
            n237 = Square Root(x=w273) -> (sqrt(x)=w272:dbl)
            n238 = Multiply(x=w272, y=1.96) -> (x*y=w264:dbl)
            n239 = Add(x=w265, y=w264) -> (x+y=w262:dbl)
            n240 = Subtract(x=w265, y=w264) -> (x-y=w263:dbl)
            n241 = Inverse Tangent(1:w262) -> (0:w260:dbl)
            n242 = Inverse Tangent(1:w263) -> (0:w259:dbl)
            n243 = Multiply(x=w260, y=w261) -> (x*y=w258:dbl)
            n244 = Multiply(x=w259, y=w261) -> (x*y=w257:dbl)
            n245 = Subtract(x=w257, y=w256) -> (x-y=w254:dbl)
            n246 = Subtract(x=w258, y=w256) -> (x-y=w255:dbl)
            n247 = Absolute Value(x=w254) -> (abs(x)=w252:dbl)
            n248 = Absolute Value(x=w255) -> (abs(x)=w253:dbl)
            n249 = Add(x=w253, y=w252) -> (x+y=w251:dbl)
            n250 = Divide(x=w251, y=2.0) -> (x/y=→"Angle Error":dbl)
          }
        }
      }
    }
    n251 = Not(x="stop") -> (.not. x?=w11:bool)
  }
  n252 = Request Deallocation(FALSE ("flag")) -> ()
